vi "grafos.vi"() -> ()   [LabVIEW 2020]
uses:
  <vilib>/measure/NI_MABase.lvlib
panel:
  out "Cuadrada":waveform(dbl)(graph)
  out "diente sierra":waveform(dbl)(graph)
  out "triangular":waveform(dbl)(graph)
  out "Senosoidal":waveform(dbl)(graph)
  in  "Frecuencia":dbl(knob) scale=0.0..60.0
  in  "Amplitud":dbl(knob) scale=0.0..220.0
  in  "stop":bool
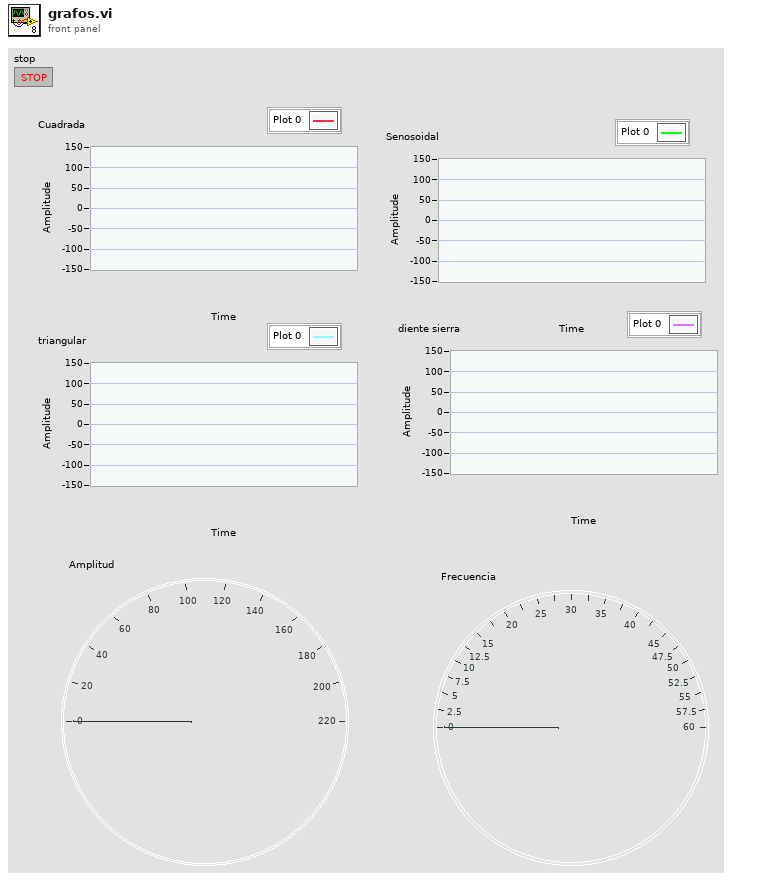
[diagram p1: front panel]
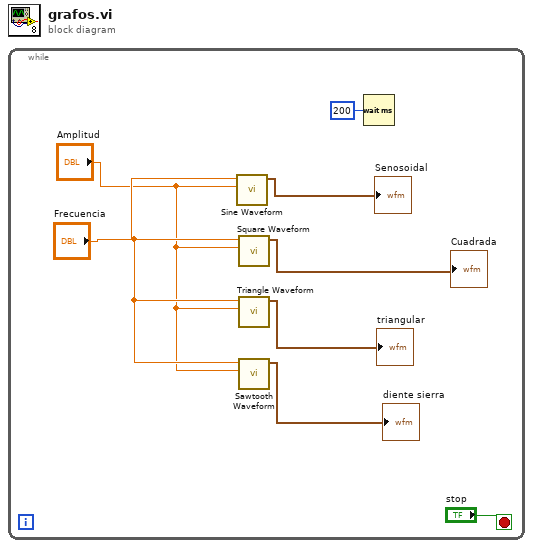
[diagram p0: block diagram]
diagram:
  n1 = while {
    stop <- "stop" stop-if-true
    n2 = call <vilib>:"Sine Waveform.vi"("amplitude"="Amplitud", "frequency"="Frecuencia") -> ("signal out"=→"Senosoidal":waveform(dbl))  [unwired: 8 in, 1 out]
    n3 = call <vilib>:"Square Waveform.vi"("amplitude"="Amplitud", "frequency"="Frecuencia") -> ("signal out"=→"Cuadrada":waveform(dbl))  [unwired: 8 in, 1 out]
    n4 = call <vilib>:"Triangle Waveform.vi"("amplitude"="Amplitud", "frequency"="Frecuencia") -> ("signal out"=→"triangular":waveform(dbl))  [unwired: 8 in, 1 out]
    n5 = call <vilib>:"Sawtooth Waveform.vi"("amplitude"="Amplitud", "frequency"="Frecuencia") -> ("signal out"=→"diente sierra":waveform(dbl))  [unwired: 8 in, 1 out]
    n6 = Wait (ms)(milliseconds to wait=u32 200) -> ()  [unwired: 1 out]
  }
